vi "Configure Triggered Value.vi"(8 "error in (no error)":errorcluster, 9 "Triggered Value (0)":dbl min=0.0 step=0.1 format="%^#_6g", 10 "Operation Mode (0: Current)":u16(ring) items=["Current", "Voltage", "Resistance", "Power"], 11 "VISA resource name":refnum<visa-resource-name>) -> (0 "error out":errorcluster, 3 "VISA resource name out":refnum<visa-resource-name>)   [LabVIEW 2017, in "HH PLI Series.lvlib"]
doc: "Sets a new setting value to the specified operation mode. The new setting value is activated after a trigger event occurred.\n\n<B>Note</B>\nTo switch into an operation mode use VI Configure Setting Value."
uses:
  HH PLI Series.lvlib
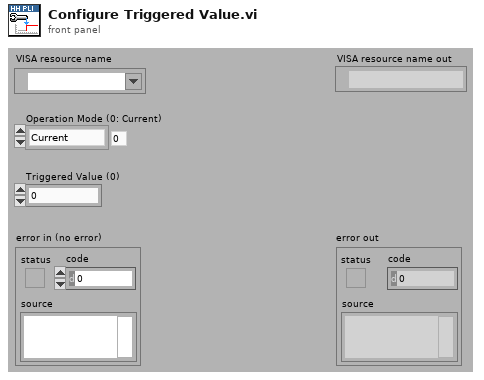
[diagram p1: front panel]
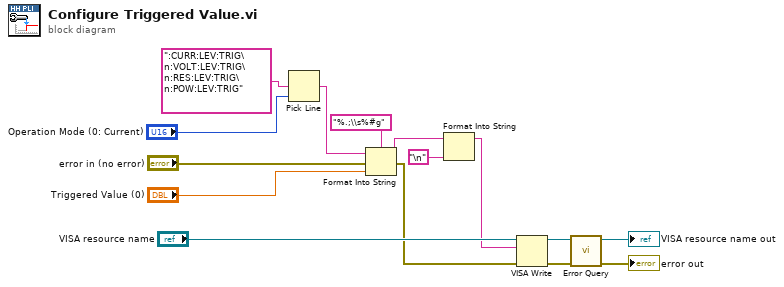
[diagram p0: block diagram]
diagram:
  n1 = Pick Line(multi-line string=":CURR:LEV:TRIG\n:VOLT:LEV:TRIG\n:RES:LEV:TRIG\n:POW:LEV:TRIG", line index="Operation Mode (0: Current)") -> (output string=w9:string)  [unwired: 1 in]
  n2 = Format Into String(format string="%.;\\s%#g", initial string=w9, error in="error in (no error)", "Triggered Value (0)") -> (resulting string=w2:string, error out=w12:errorcluster)
  n3 = Format Into String(initial string=w2, "\n") -> (resulting string=w1:string)  [unwired: 2 in, 1 out]
  n4 = VISA Write(VISA resource name="VISA resource name", write buffer=w1, error in (no error)=w12) -> (VISA resource name out=w7:refnum<visa-resource-name>, error out=w8:errorcluster)  [unwired: 1 out]
  n5 = call "Error Query.vi"("error in (no error)"=w8, "VISA resource name"=w7) -> ("error out"=→"error out":errorcluster, "VISA resource name out"=→"VISA resource name out":refnum<visa-resource-name>)  [unwired: 6 in, 2 out]
